vi "PullPush.vi"(6 "speed_uL_s":dbl, 7 "pushTo":string, 9 "volume_uL":dbl, 10 "pullFrom":string, 11 ".NET Refnum in":refnum<k24>) -> (3 ".NET Refnum out":refnum<k24>)   [LabVIEW 2020]
uses:
  D:/PumpAutomation2/DEMPBot2/PumpAdapter.exe
  PumpAdapter.exe
panel:
  out "PullPush":string
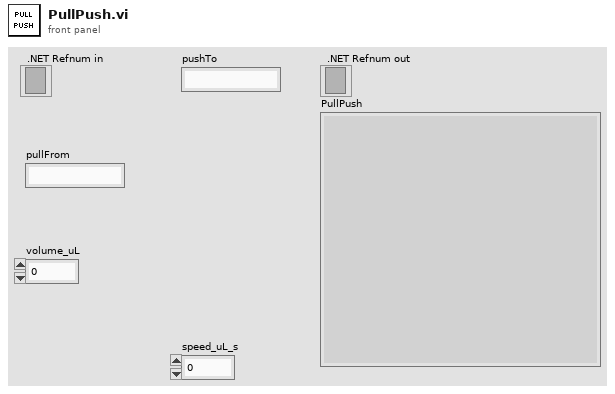
[diagram p1: front panel]
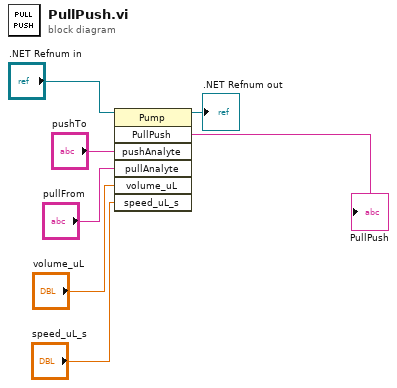
[diagram p0: block diagram]
diagram:
  n1 = invoke class="Pump" method="PullPush"(reference=".NET Refnum in", "pushAnalyte"="pushTo", "pullAnalyte"="pullFrom", "volume_uL"="volume_uL", "speed_uL_s"="speed_uL_s") -> (reference out=→".NET Refnum out":refnum<k24>, "PullPush"=→"PullPush":string)  [unwired: 2 in, 5 out]
